vi "Client References Parse Command.vi"(11 "Queue Command (\"\")":string) -> (2 "Params":string[](array[string]), 3 "Function":string, 5 "HTTP Port":u16)   [LabVIEW 2011]
uses:
  Spartan Client Version.vi
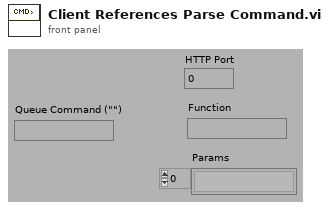
[diagram p1: front panel]
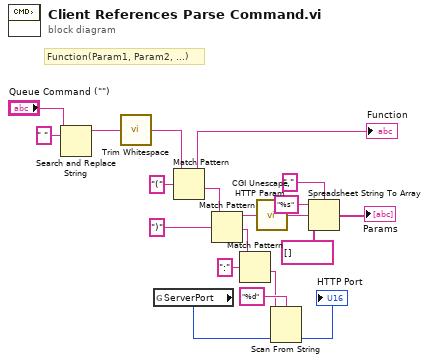
[diagram p0: block diagram]
diagram:
  # "Function(Param1, Param2, ...)"
  n1 = Search and Replace String(input string="Queue Command (\"\")", search string=" ") -> (result string=w10:string)  [unwired: 1 in, 8 out]
  n2 = call <vilib>:"Trim Whitespace.vi"("string"=w10) -> ("trimmed string"=w8:string)  [unwired: 1 in]
  n3 = global read "Spartan Client Version.vi" "ServerPort"() -> (w2:u16)
  n4 = Match Pattern(string=w8, regular expression="(") -> (before substring=→"Function":string, after substring=w18:string)  [unwired: 3 out]
  n5 = Match Pattern(string=w18, regular expression=")") -> (before substring=w16:string, after substring=w5:string)  [unwired: 3 out]
  n6 = Match Pattern(string=w5, regular expression=":") -> (after substring=w3:string)  [unwired: 4 out]
  n7 = call "CGI Unescape HTTP Param.vi"("url-encoded string"=w16) -> ("string"=w7:string)
  n8 = Scan From String(format string="%d", input string=w3, default 1=w2) -> (output 1=→"HTTP Port":u16)  [unwired: 2 in, 3 out]
  n9 = Spreadsheet String To Array(delimiter (Tab)=",", format string="%s", spreadsheet string=w7, array type (2D Dbl)=string[] []) -> (array=→"Params":string[])
